vi "获取最新数据的日期.vi"(8 "error in (no error)":errorcluster, 10 "表名":string, 11 "数据库连接引用 i":T1) -> (0 "error out":errorcluster, 1 "报警？":bool, 2 "累积值":dbl, 3 "数据库连接引用 o":T1, 5 "起始时间":timestamp)   [LabVIEW 2017]
uses:
  <vilib>/addons/database/Connection.llb/Conn ObjectReference.ctl
  <vilib>/addons/database/NI_Database_API.lvlib
panel:
  out "字符串数据":string[][](array[string])
  out "Result":string caption="结果"
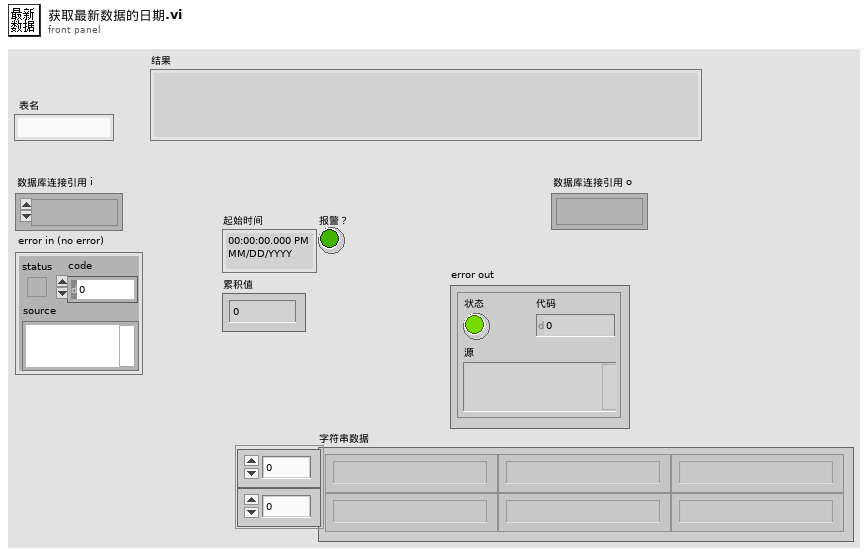
[diagram p1: front panel]
types:
  T1 = typedef "NI_Database_API.lvlib/Conn ObjectReference.ctl" = refnum<k1>
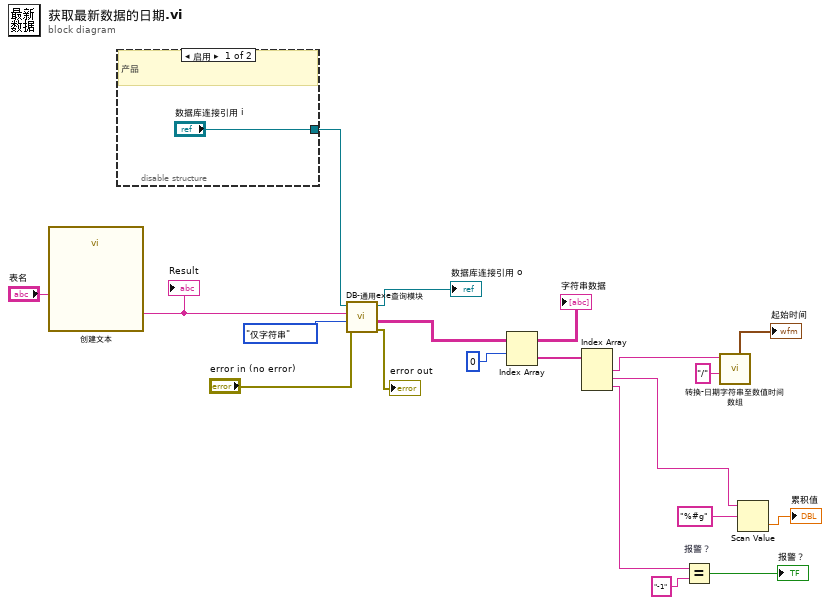
[diagram p0: block diagram]
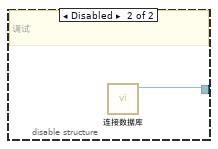
[diagram p2: hidden frame]
diagram:
  n1 = call "创建文本"("表名"="表名") -> ("Result"=w4:string)  [unwired: 13 in, 1 out]
  "Result" <- w4
  n2 = disable-structure shown="启用" {
    disable-tunnel: ["数据库连接引用 i" w21] -> w14
    frame Enabled {
      # "产品"
    }
    frame Disabled {
      # "调试"
      n3 = call "连接数据库.vi"() -> ("connection reference"=w21:T1)  [unwired: 10 in, 1 out]
    }
  }
  n4 = call "DB-通用exe查询模块.vi"("error in (no error)"="error in (no error)", "解析模式"=enum16{"仅数值", "仅字符串", "数值与字符串"}."仅字符串", "SQL query"=w4, "数据库连接引用"=w14) -> ("error out"=→"error out":errorcluster, "字符串数据"=w19:string[][], "数据库连接引用out"=→"数据库连接引用 o":T1)  [unwired: 3 in, 2 out]
  "字符串数据" <- w19
  n5 = Index Array(array=w19, index (row)=0 ("禁用的索引 (列)")) -> (element=w12:string[])  [unwired: 1 in]
  n6 = Index Array(array=w12) -> (element #1=w11:string, element #2=w2:string, element #3=w9:string)  [unwired: 3 in]
  n7 = Equal? "报警？"(x=w9, y="-1") -> (x = y?=→"报警？":bool)
  n8 = call "转换-日期字符串至数值时间数组.vi"("分隔符（/）"="/", "日期时间（或仅日期）字符串"=w11) -> ("时间标识"=→"起始时间":timestamp)  [unwired: 5 in, 4 out]
  n9 = Scan Value(string=w2, format string="%#g" ("格式字符串")) -> (value=→"累积值":dbl)  [unwired: 1 in, 1 out]
